vi "Active Project Scope Index.vi"(8 "Error In":errorcluster, 10 "Strings[]":string[](array[string]), 11 "App In":refnum<vi>) -> (0 "Error Out":errorcluster, 2 "Index":i32=-1, 3 "App Out":refnum<vi>)   [LabVIEW 2017, in "Bookmark Manager.lvlib"]
doc: "Determines which project to use for the scope from the list of projects that will be used for the scope's ring."
uses:
  Bookmark Manager.lvlib
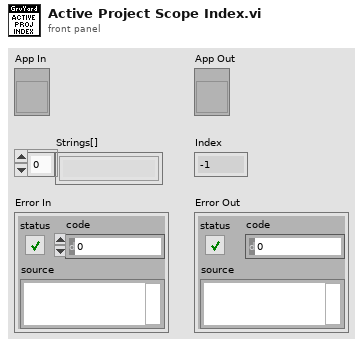
[diagram p1: front panel]
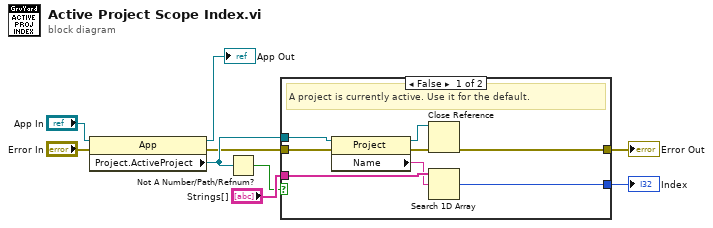
[diagram p0: block diagram]
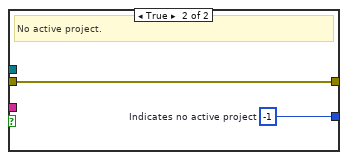
[diagram p2: hidden frame]
diagram:
  n1 = property class="App"(reference="App In", error in="Error In") -> (reference out=→"App Out":refnum<vi>, error out=w6:errorcluster, "Project.ActiveProject"=w7:refnum<vi>)
  n2 = Not A Number/Path/Refnum?(number/path/refnum=w7) -> (NaN/Path/Refnum?=w5:bool)
  n3 = case shown="False" w5 {
    tunnel: w6 -> [w16 w19]
    tunnel: w7 -> [w17 _]
    tunnel: [w13 w19] -> w8
    tunnel: "Strings[]" -> [w12 _]
    tunnel: [w10 w18] -> w1
    frame False {
      # "A project is currently active. Use it for the default."
      n4 = property class="Project"(reference=w17, error in=w16) -> (reference out=w15:refnum<vi>, error out=w14:errorcluster, "Name"=w11:string)
      n5 = Close Reference(reference=w15, error in (no error)=w14) -> (error out=w13:errorcluster)
      n6 = Search 1D Array(1D array=w12, element=w11) -> (index of element=w10:i32)  [unwired: 1 in]
    }
    frame True {
      w18 = -1  # Indicates no active project
      # "No active project."
    }
  }
  "Error Out" <- w8
  "Index" <- w1
